vi "VISJS Viewer.vi"(4 "Extra Scripts":string, 5 "FileDependency In":map{path, T1}(c390), 6 "Options":string, 7 "OpenWebBrowser(False)":bool, 8 "error in":errorcluster, 9 "Embedd VISJS Librarya in HTMl File(False)":bool, 10 "HTMLFilePath":path, 11 "LibraryDependency":map{path, T3}(c390)) -> (0 "error out":errorcluster, 3 "HTMLFileContent":string)   [LabVIEW 2020, in "VISJS Viewer.lvlib"] (continued)
this.frame.appendChild(this.opacityDiv),this.frame.appendChild(this.newColorDiv),this.frame.appendChild(this.initialColorDiv),this.frame.appendChild(this.cancelButton),this.frame.appendChild(this.applyButton),this.frame.appendChild(this.saveButton),this.frame.appendChild(this.loadButton)}},{key:\"_bindHammer\",value:function(){var g=this;this.drag={},this.pinch={},this.hammer=new Gf(this.colorPickerCanvas),this.hammer.get(\"pinch\").set({enable:!0}),this.hammer.on(\"hammer.input\",(function(t){t.isFirst&&g._moveSelector(t)})),this.hammer.on(\"tap\",(function(t){g._moveSelector(t)})),this.hammer.on(\"panstart\",(function(t){g._moveSelector(t)})),this.hammer.on(\"panmove\",(function(t){g._moveSelector(t)})),this.hammer.on(\"panend\",(function(t){g._moveSelector(t)}))}},{key:\"_generateHueCircle\",value:function(){if(!1===this.generated){var g=this.colorPickerCanvas.getContext(\"2d\");void 0===this.pixelRation&&(this.pixelRatio=(window.devicePixelRatio||1)/(g.webkitBackingStorePixelRatio||g.mozBackingStorePixelRatio||g.msBackingStorePixelRatio||g.oBackingStorePixelRatio||g.backingStorePixelRatio||1)),g.setTransform(this.pixelRatio,0,0,this.pixelRatio,0,0);var t,A,e,C,I=this.colorPickerCanvas.clientWidth,i=this.colorPickerCanvas.clientHeight;g.clearRect(0,0,I,i),this.centerCoordinates={x:.5*I,y:.5*i},this.r=.49*I;var o,n=2*Math.PI/360,r=1/this.r;for(e=0;e<360;e++)for(C=0;C<this.r;C++)t=this.centerCoordinates.x+C*Math.sin(n*e),A=this.centerCoordinates.y+C*Math.cos(n*e),o=ov(.002777777777777778*e,C*r,1),g.fillStyle=\"rgb(\"+o.r+\",\"+o.g+\",\"+o.b+\")\",g.fillRect(t-.5,A-.5,2,2);g.strokeStyle=\"rgba(0,0,0,1)\",g.circle(this.centerCoordinates.x,this.centerCoordinates.y,this.r),g.stroke(),this.hueCircle=g.getImageData(0,0,I,i)}this.generated=!0}},{key:\"_moveSelector\",value:function(g){var t=this.colorPickerDiv.getBoundingClientRect(),A=g.center.x-t.left,e=g.center.y-t.top,C=.5*this.colorPickerDiv.clientHeight,I=.5*this.colorPickerDiv.clientWidth,i=A-I,o=e-C,n=Math.atan2(i,o),r=.98*Math.min(Math.sqrt(i*i+o*o),I),s=Math.cos(n)*r+C,a=Math.sin(n)*r+I;this.colorPickerSelector.style.top=s-.5*this.colorPickerSelector.clientHeight+\"px\",this.colorPickerSelector.style.left=a-.5*this.colorPickerSelector.clientWidth+\"px\";var d=n/(2*Math.PI);d=d<0?d+1:d;var h=r/this.r,l=iv(this.color.r,this.color.g,this.color.b);l.h=d,l.s=h;var c=ov(l.h,l.s,l.v);c.a=this.color.a,this.color=c,this.initialColorDiv.style.backgroundColor=\"rgba(\"+this.initialColor.r+\",\"+this.initialColor.g+\",\"+this.initialColor.b+\",\"+this.initialColor.a+\")\",this.newColorDiv.style.backgroundColor=\"rgba(\"+this.color.r+\",\"+this.color.g+\",\"+this.color.b+\",\"+this.color.a+\")\"}}]),g}();function pv(){for(var g=arguments.length,t=new Array(g),A=0;A<g;A++)t[A]=arguments[A];if(t.length<1)throw new TypeError(\"Invalid arguments.\");if(1===t.length)return document.createTextNode(t[0]);var e=document.createElement(t[0]);return e.appendChild(pv.apply(void 0,ch(wh(t).call(t,1)))),e}var fv,vv=function(){function g(t,A,e){var C=arguments.length>3&&void 0!==arguments[3]?arguments[3]:1,I=arguments.length>4&&void 0!==arguments[4]?arguments[4]:function(){return!1};cn(this,g),this.parent=t,this.changedOptions=[],this.container=A,this.allowCreation=!1,this.hideOption=I,this.options={},this.initialized=!1,this.popupCounter=0,this.defaultOptions={enabled:!1,filter:!0,container:void 0,showButton:!0},fe(this.options,this.defaultOptions),this.configureOptions=e,this.moduleOptions={},this.domElements=[],this.popupDiv={},this.popupLimit=5,this.popupHistory={},this.colorPicker=new uv(C),this.wrapper=void 0}return kd(g,[{key:\"setOptions\",value:function(g){if(void 0!==g){this.popupHistory={},this._removePopup();var t=!0;if(\"string\"==typeof g)this.options.filter=g;else if(Rh(g))this.options.filter=g.join();else if(\"object\"===yd(g)){if(null==g)throw new TypeError(\"options cannot be null\");void 0!==g.container&&(this.options.container=g.container),void 0!==pc(g)&&(this.options.filter=pc(g)),void 0!==g.showButton&&(this.options.showButton=g.showButton),void 0!==g.enabled&&(t=g.enabled)}else\"boolean\"==typeof g?(this.options.filter=!0,t=g):\"function\"==typeof g&&(this.options.filter=g,t=!0);!1===pc(this.options)&&(t=!1),this.options.enabled=t}this._clean()}},{key:\"setModuleOptions\",value:function(g){this.moduleOptions=g,!0===this.options.enabled&&(this._clean(),void 0!==this.options.container&&(this.container=this.options.container),this._create())}},{key:\"_create\",value:function(){this._clean(),this.changedOptions=[];var g=pc(this.options),t=0,A=!1;for(var e in this.configureOptions)Object.prototype.hasOwnProperty.call(this.configureOptions,e)&&(this.allowCreation=!1,A=!1,\"function\"==typeof g?A=(A=g(e,[]))||this._handleObject(this.configureOptions[e],[e],!0):!0!==g&&-1===Xc(g).call(g,e)||(A=!0),!1!==A&&(this.allowCreation=!0,t>0&&this._makeItem([]),this._makeHeader(e),this._handleObject(this.configureOptions[e],[e])),t++);this._makeButton(),this._push()}},{key:\"_push\",value:function(){this.wrapper=document.createElement(\"div\"),this.wrapper.className=\"vis-configuration-wrapper\",this.container.appendChild(this.wrapper);for(var g=0;g<this.domElements.length;g++)this.wrapper.appendChild(this.domElements[g]);this._showPopupIfNeeded()}},{key:\"_clean\",value:function(){for(var g=0;g<this.domElements.length;g++)this.wrapper.removeChild(this.domElements[g]);void 0!==this.wrapper&&(this.container.removeChild(this.wrapper),this.wrapper=void 0),this.domElements=[],this._removePopup()}},{key:\"_getValue\",value:function(g){for(var t=this.moduleOptions,A=0;A<g.length;A++){if(void 0===t[g[A]]){t=void 0;break}t=t[g[A]]}return t}},{key:\"_makeItem\",value:function(g){if(!0===this.allowCreation){var t=document.createElement(\"div\");t.className=\"vis-configuration vis-config-item vis-config-s\"+g.length;for(var A=arguments.length,e=new Array(A>1?A-1:0),C=1;C<A;C++)e[C-1]=arguments[C];return Cl(e).call(e,(function(g){t.appendChild(g)})),this.domElements.push(t),this.domElements.length}return 0}},{key:\"_makeHeader\",value:function(g){var t=document.createElement(\"div\");t.className=\"vis-configuration vis-config-header\",t.innerText=g,this._makeItem([],t)}},{key:\"_makeLabel\",value:function(g,t){var A=arguments.length>2&&void 0!==arguments[2]&&arguments[2],e=document.createElement(\"div\");if(e.className=\"vis-configuration vis-config-label vis-config-s\"+t.length,!0===A){for(;e.firstChild;)e.removeChild(e.firstChild);e.appendChild(pv(\"i\",\"b\",g))}else e.innerText=g+\":\";return e}},{key:\"_makeDropdown\",value:function(g,t,A){var e=document.createElement(\"select\");e.className=\"vis-configuration vis-config-select\";var C=0;void 0!==t&&-1!==Xc(g).call(g,t)&&(C=Xc(g).call(g,t));for(var I=0;I<g.length;I++){var i=document.createElement(\"option\");i.value=g[I],I===C&&(i.selected=\"selected\"),i.innerText=g[I],e.appendChild(i)}var o=this;e.onchange=function(){o._update(this.value,A)};var n=this._makeLabel(A[A.length-1],A);this._makeItem(A,n,e)}},{key:\"_makeRange\",value:function(g,t,A){var e=g[0],C=g[1],I=g[2],i=g[3],o=document.createElement(\"input\");o.className=\"vis-configuration vis-config-range\";try{o.type=\"range\",o.min=C,o.max=I}catch(g){}o.step=i;var n=\"\",r=0;if(void 0!==t){var s=1.2;t<0&&t*s<C?(o.min=Math.ceil(t*s),r=o.min,n=\"range increased\"):t/s<C&&(o.min=Math.ceil(t/s),r=o.min,n=\"range increased\"),t*s>I&&1!==I&&(o.max=Math.ceil(t*s),r=o.max,n=\"range increased\"),o.value=t}else o.value=e;var a=document.createElement(\"input\");a.className=\"vis-configuration vis-config-rangeinput\",a.value=o.value;var d=this;o.onchange=function(){a.value=this.value,d._update(Number(this.value),A)},o.oninput=function(){a.value=this.value};var h=this._makeLabel(A[A.length-1],A),l=this._makeItem(A,h,o,a);\"\"!==n&&this.popupHistory[l]!==r&&(this.popupHistory[l]=r,this._setupPopup(n,l))}},{key:\"_makeButton\",value:function(){var g=this;if(!0===this.options.showButton){var t=document.createElement(\"div\");t.className=\"vis-configuration vis-config-button\",t.innerText=\"generate options\",t.onclick=function(){g._printOptions()},t.onmouseover=function(){t.className=\"vis-configuration vis-config-button hover\"},t.onmouseout=function(){t.className=\"vis-configuration vis-config-button\"},this.optionsContainer=document.createElement(\"div\"),this.optionsContainer.className=\"vis-configuration vis-config-option-container\",this.domElements.push(this.optionsContainer),this.domElements.push(t)}}},{key:\"_setupPopup\",value:function(g,t){var A=this;if(!0===this.initialized&&!0===this.allowCreation&&this.popupCounter<this.popupLimit){var e=document.createElement(\"div\");e.id=\"vis-configuration-popup\",e.className=\"vis-configuration-popup\",e.innerText=g,e.onclick=function(){A._removePopup()},this.popupCounter+=1,this.popupDiv={html:e,index:t}}}},{key:\"_removePopup\",value:function(){void 0!==this.popupDiv.html&&(this.popupDiv.html.parentNode.removeChild(this.popupDiv.html),clearTimeout(this.popupDiv.hideTimeout),clearTimeout(this.popupDiv.deleteTimeout),this.popupDiv={})}},{key:\"_showPopupIfNeeded\",value:function(){var g=this;if(void 0!==this.popupDiv.html){var t=this.domElements[this.popupDiv.index].getBoundingClientRect();this.popupDiv.html.style.left=t.left+\"px\",this.popupDiv.html.style.top=t.top-30+\"px\",document.body.appendChild(this.popupDiv.html),this.popupDiv.hideTimeout=wu((function(){g.popupDiv.html.style.opacity=0}),1500),this.popupDiv.deleteTimeout=wu((function(){g._removePopup()}),1800)}}},{key:\"_makeCheckbox\",value:function(g,t,A){var e=document.createElement(\"input\");e.type=\"checkbox\",e.className=\"vis-configuration vis-config-checkbox\",e.checked=g,void 0!==t&&(e.checked=t,t!==g&&(\"object\"===yd(g)?t!==g.enabled&&this.changedOptions.push({path:A,value:t}):this.changedOptions.push({path:A,value:t})));var C=this;e.onchange=function(){C._update(this.checked,A)};var I=this._makeLabel(A[A.length-1],A);this._makeItem(A,I,e)}},{key:\"_makeTextInput\",value:function(g,t,A){var e=document.createElement(\"input\");e.type=\"text\",e.className=\"vis-configuration vis-config-text\",e.value=t,t!==g&&this.changedOptions.push({path:A,value:t});var C=this;e.onchange=function(){C._update(this.value,A)};var I=this._makeLabel(A[A.length-1],A);this._makeItem(A,I,e)}},{key:\"_makeColorField\",value:function(g,t,A){var e=this,C=g[1],I=document.createElement(\"div\");\"none\"!==(t=void 0===t?C:t)?(I.className=\"vis-configuration vis-config-colorBlock\",I.style.backgroundColor=t):I.className=\"vis-configuration vis-config-colorBlock none\",t=void 0===t?C:t,I.onclick=function(){e._showColorPicker(t,I,A)};var i=this._makeLabel(A[A.length-1],A);this._makeItem(A,i,I)}},{key:\"_showColorPicker\",value:function(g,t,A){var e=this;t.onclick=function(){},this.colorPicker.insertTo(t),this.colorPicker.show(),this.colorPicker.setColor(g),this.colorPicker.setUpdateCallback((function(g){var C=\"rgba(\"+g.r+\",\"+g.g+\",\"+g.b+\",\"+g.a+\")\";t.style.backgroundColor=C,e._update(C,A)})),this.colorPicker.setCloseCallback((function(){t.onclick=function(){e._showColorPicker(g,t,A)}}))}},{key:\"_handleObject\",value:function(g){var t=arguments.length>1&&void 0!==arguments[1]?arguments[1]:[],A=arguments.length>2&&void 0!==arguments[2]&&arguments[2],e=!1,C=pc(this.options),I=!1;for(var i in g)if(Object.prototype.hasOwnProperty.call(g,i)){e=!0;var o=g[i],n=$f(t,i);if(\"function\"==typeof C&&!1===(e=C(i,t))&&!Rh(o)&&\"string\"!=typeof o&&\"boolean\"!=typeof o&&o instanceof Object&&(this.allowCreation=!1,e=this._handleObject(o,n,!0),this.allowCreation=!1===A),!1!==e){I=!0;var r=this._getValue(n);if(Rh(o))this._handleArray(o,r,n);else if(\"string\"==typeof o)this._makeTextInput(o,r,n);else if(\"boolean\"==typeof o)this._makeCheckbox(o,r,n);else if(o instanceof Object){if(!this.hideOption(t,i,this.moduleOptions))if(void 0!==o.enabled){var s=$f(n,\"enabled\"),a=this._getValue(s);if(!0===a){var d=this._makeLabel(i,n,!0);this._makeItem(n,d),I=this._handleObject(o,n)||I}else this._makeCheckbox(o,a,n)}else{var h=this._makeLabel(i,n,!0);this._makeItem(n,h),I=this._handleObject(o,n)||I}}else console.error(\"dont know how to handle\",o,i,n)}}return I}},{key:\"_handleArray\",value:function(g,t,A){\"string\"==typeof g[0]&&\"color\"===g[0]?(this._makeColorField(g,t,A),g[1]!==t&&this.changedOptions.push({path:A,value:t})):\"string\"==typeof g[0]?(this._makeDropdown(g,t,A),g[0]!==t&&this.changedOptions.push({path:A,value:t})):\"number\"==typeof g[0]&&(this._makeRange(g,t,A),g[0]!==t&&this.changedOptions.push({path:A,value:Number(t)}))}},{key:\"_update\",value:function(g,t){var A=this._constructOptions(g,t);this.parent.body&&this.parent.body.emitter&&this.parent.body.emitter.emit&&this.parent.body.emitter.emit(\"configChange\",A),this.initialized=!0,this.parent.setOptions(A)}},{key:\"_constructOptions\",value:function(g,t){var A=arguments.length>2&&void 0!==arguments[2]?arguments[2]:{},e=A;g=\"false\"!==(g=\"true\"===g||g)&&g;for(var C=0;C<t.length;C++)\"global\"!==t[C]&&(void 0===e[t[C]]&&(e[t[C]]={}),C!==t.length-1?e=e[t[C]]:e[t[C]]=g);return A}},{key:\"_printOptions\",value:function(){for(var g=this.getOptions();this.optionsContainer.firstChild;)this.optionsContainer.removeChild(this.optionsContainer.firstChild);this.optionsContainer.appendChild(pv(\"pre\",\"const options = \"+eu(g,null,2)))}},{key:\"getOptions\",value:function(){for(var g={},t=0;t<this.changedOptions.length;t++)this._constructOptions(this.changedOptions[t].value,this.changedOptions[t].path,g);return g}}]),g}(),yv=function(){function g(t,A){cn(this,g),this.container=t,this.overflowMethod=A||\"cap\",this.x=0,this.y=0,this.padding=5,this.hidden=!1,this.frame=document.createElement(\"div\"),this.frame.className=\"vis-tooltip\",this.container.appendChild(this.frame)}return kd(g,[{key:\"setPosition\",value:function(g,t){this.x=Gc(g),this.y=Gc(t)}},{key:\"setText\",value:function(g){if(g instanceof Element){for(;this.frame.firstChild;)this.frame.removeChild(this.frame.firstChild);this.frame.appendChild(g)}else this.frame.innerText=g}},{key:\"show\",value:function(g){if(void 0===g&&(g=!0),!0===g){var t=this.frame.clientHeight,A=this.frame.clientWidth,e=this.frame.parentNode.clientHeight,C=this.frame.parentNode.clientWidth,I=0,i=0;if(\"flip\"==this.overflowMethod){var o=!1,n=!0;this.y-t<this.padding&&(n=!1),this.x+A>C-this.padding&&(o=!0),I=o?this.x-A:this.x,i=n?this.y-t:this.y}else(i=this.y-t)+t+this.padding>e&&(i=e-t-this.padding),i<this.padding&&(i=this.padding),(I=this.x)+A+this.padding>C&&(I=C-A-this.padding),I<this.padding&&(I=this.padding);this.frame.style.left=I+\"px\",this.frame.style.top=i+\"px\",this.frame.style.visibility=\"visible\",this.hidden=!1}else this.hide()}},{key:\"hide\",value:function(){this.hidden=!0,this.frame.style.left=\"0\",this.frame.style.top=\"0\",this.frame.style.visibility=\"hidden\"}},{key:\"destroy\",value:function(){this.frame.parentNode.removeChild(this.frame)}}]),g}(),mv=!1,bv=\"background: #FFeeee; color: #dd0000\",wv=function(){function g(){cn(this,g)}return kd(g,null,[{key:\"validate\",value:function(t,A,e){mv=!1,fv=A;var C=A;return void 0!==e&&(C=A[e]),g.parse(t,C,[]),mv}},{key:\"parse\",value:function(t,A,e){for(var C in t)Object.prototype.hasOwnProperty.call(t,C)&&g.check(C,t,A,e)}},{key:\"check\",value:function(t,A,e,C){if(void 0!==e[t]||void 0!==e.__any__){var I=t,i=!0;void 0===e[t]&&void 0!==e.__any__&&(I=\"__any__\",i=\"object\"===g.getType(A[t]));var o=e[I];i&&void 0!==o.__type__&&(o=o.__type__),g.checkFields(t,A,e,I,o,C)}else g.getSuggestion(t,e,C)}},{key:\"checkFields\",value:function(t,A,e,C,I,i){var o=function(A){console.error(\"%c\"+A+g.printLocation(i,t),bv)},n=g.getType(A[t]),r=I[n];void 0!==r?\"array\"===g.getType(r)&&-1===Xc(r).call(r,A[t])?(o('Invalid option detected in \"'+t+'\". Allowed values are:'+g.print(r)+' not \"'+A[t]+'\". '),mv=!0):\"object\"===n&&\"__any__\"!==C&&(i=$f(i,t),g.parse(A[t],e[C],i)):void 0===I.any&&(o('Invalid type received for \"'+t+'\". Expected: '+g.print(Lh(I))+\". Received [\"+n+'] \"'+A[t]+'\"'),mv=!0)}},{key:\"getType\",value:function(g){var t=yd(g);return\"object\"===t?null===g?\"null\":g instanceof Boolean?\"boolean\":g instanceof Number?\"number\":g instanceof String?\"string\":Rh(g)?\"array\":g instanceof Date?\"date\":void 0!==g.nodeType?\"dom\":!0===g._isAMomentObject?\"moment\":\"object\":\"number\"===t?\"number\":\"boolean\"===t?\"boolean\":\"string\"===t?\"string\":void 0===t?\"undefined\":t}},{key:\"getSuggestion\",value:function(t,A,e){var C,I=g.findInOptions(t,A,e,!1),i=g.findInOptions(t,fv,[],!0);C=void 0!==I.indexMatch?\" in \"+g.printLocation(I.path,t,\"\")+'Perhaps it was incomplete? Did you mean: \"'+I.indexMatch+'\"?\\n\\n':i.distance<=4&&I.distance>i.distance?\" in \"+g.printLocation(I.path,t,\"\")+\"Perhaps it was misplaced? Matching option found at: \"+g.printLocation(i.path,i.closestMatch,\"\"):I.distance<=8?'. Did you mean \"'+I.closestMatch+'\"?'+g.printLocation(I.path,t):\". Did you mean one of these: \"+g.print(Lh(A))+g.printLocation(e,t),console.error('%cUnknown option detected: \"'+t+'\"'+C,bv),mv=!0}},{key:\"findInOptions\",value:function(t,A,e){var C,I=arguments.length>3&&void 0!==arguments[3]&&arguments[3],i=1e9,o=\"\",n=[],r=t.toLowerCase(),s=void 0;for(var a in A){var d=void 0;if(void 0!==A[a].__type__&&!0===I){var h=g.findInOptions(t,A[a],$f(e,a));i>h.distance&&(o=h.closestMatch,n=h.path,i=h.distance,s=h.indexMatch)}else{var l;-1!==Xc(l=a.toLowerCase()).call(l,r)&&(s=a),i>(d=g.levenshteinDistance(t,a))&&(o=a,n=wh(C=e).call(C),i=d)}}return{closestMatch:o,path:n,distance:i,indexMatch:s}}},{key:\"printLocation\",value:function(g,t){for(var A=\"\\n\\n\"+(arguments.length>2&&void 0!==arguments[2]?arguments[2]:\"Problem value found at: \\n\")+\"options = {\\n\",e=0;e<g.length;e++){for(var C=0;C<e+1;C++)A+=\"  \";A+=g[e]+\": {\\n\"}for(var I=0;I<g.length+1;I++)A+=\"  \";A+=t+\"\\n\";for(var i=0;i<g.length+1;i++){for(var o=0;o<g.length-i;o++)A+=\"  \";A+=\"}\\n\"}return A+\"\\n\\n\"}},{key:\"print\",value:function(g){return eu(g).replace(/(\")|(\\[)|(\\])|(,\"__type__\")/g,\"\").replace(/(,)/g,\", \")}},{key:\"levenshteinDistance\",value:function(g,t){if(0===g.length)return t.length;if(0===t.length)return g.length;var A,e,C=[];for(A=0;A<=t.length;A++)C[A]=[A];for(e=0;e<=g.length;e++)C[0][e]=e;for(A=1;A<=t.length;A++)for(e=1;e<=g.length;e++)t.charAt(A-1)==g.charAt(e-1)?C[A][e]=C[A-1][e-1]:C[A][e]=Math.min(C[A-1][e-1]+1,Math.min(C[A][e-1]+1,C[A-1][e]+1));return C[t.length][g.length]}}]),g}(),kv=jf,xv=vv,Ev=Gf,Ov=yv,Tv=bv,Dv=wv;function Nv(g){return zv=g,function(){var g={};Sv=0,void(Zv=zv.charAt(0)),Kv(),\"strict\"===Fv&&(g.strict=!0,Kv());\"graph\"!==Fv&&\"digraph\"!==Fv||(g.type=Fv,Kv());Gv===Mv.IDENTIFIER&&(g.id=Fv,Kv());if(\"{\"!=Fv)throw gy(\"Angle bracket { expected\");if(Kv(),Hv(g),\"}\"!=Fv)throw gy(\"Angle bracket } expected\");if(Kv(),\"\"!==Fv)throw gy(\"End of file expected\");return Kv(),delete g.node,delete g.edge,delete g.graph,g}()}var Rv={fontsize:\"font.size\",fontcolor:\"font.color\",labelfontcolor:\"font.color\",fontname:\"font.face\",color:[\"color.border\",\"color.background\"],fillcolor:\"color.background\",tooltip:\"title\",labeltooltip:\"title\"},Pv=$c(Rv);Pv.color=\"color.color\",Pv.style=\"dashes\";var Mv={NULL:0,DELIMITER:1,IDENTIFIER:2,UNKNOWN:3},Bv={\"{\":!0,\"}\":!0,\"[\":!0,\"]\":!0,\";\":!0,\"=\":!0,\",\":!0,\"->\":!0,\"--\":!0},zv=\"\",Sv=0,Zv=\"\",Fv=\"\",Gv=Mv.NULL;function jv(){Sv++,Zv=zv.charAt(Sv)}function Lv(){return zv.charAt(Sv+1)}function Vv(g){var t=g.charCodeAt(0);return t<47?35===t||46===t:t<59?t>47:t<91?t>64:t<96?95===t:t<123&&t>96}function Yv(g,t){if(g||(g={}),t)for(var A in t)t.hasOwnProperty(A)&&(g[A]=t[A]);return g}function Wv(g,t,A){for(var e=t.split(\".\"),C=g;e.length;){var I=e.shift();e.length?(C[I]||(C[I]={}),C=C[I]):C[I]=A}}function Qv(g,t){for(var A,e,C=null,I=[g],i=g;i.parent;)I.push(i.parent),i=i.parent;if(i.nodes)for(A=0,e=i.nodes.length;A<e;A++)if(t.id===i.nodes[A].id){C=i.nodes[A];
